vi "DEMO_01_SER-2014.vi"() -> ()   [LabVIEW 2014]
uses:
  <vilib>/Instr/_visa.llb/VISA Configure Serial Port (Instr).vi
panel:
  in  "开闭环":u16(ring) items=["  开环", "  闭环"]
  in  "通道":enum16{"  一路", "  二路", "  三路"}(ring)
  in  "发送数据":dbl
  out "添加的数组":i32[](array[numeric])
  out "抑或后的数据值":u8
  in  "stop":bool
  in  "退出":bool
  in  "发送":bool
  in  "上位机控制":bool
  in  "VISA资源名称":refnum<visa-resource-name>="COM1"
  in  "波特率":u32(ring)=9600 items=["75"=75, "110"=110, "134"=134, "150"=150, "300"=300, "600"=600, "1200"=1200, "1800"=1800, "2400"=2400, "4800"=4800, "7200"=7200, "9600"=9600, "14400"=14400, "19200"=19200, "28800"=28800, "38400"=38400, "56000"=56000, "57600"=57600, "115200"=115200, "128000"=128000, "230400"=230400]
  in  "奇偶":enum16{"None", "Odd", "Even", "Mark", "Space"}(ring) caption="校验"
  # "哈尔滨芯明天科技labview例程发送单点数据"
  # "测试的数组"
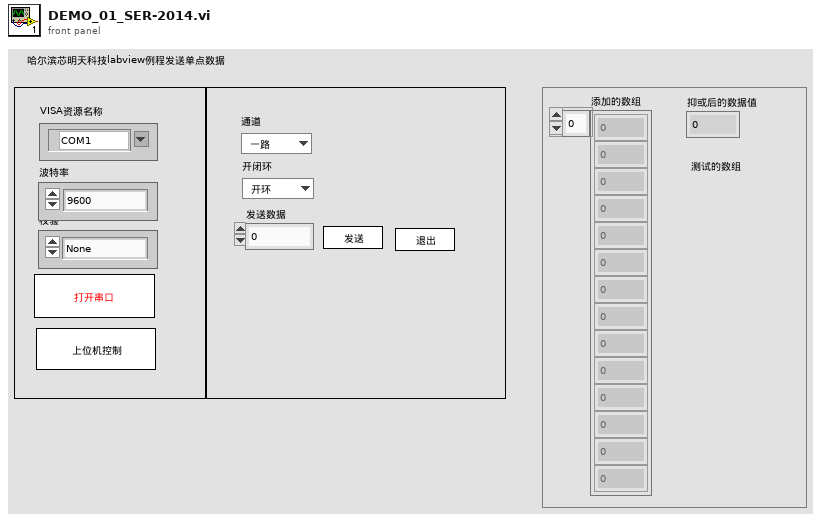
[diagram p1: front panel]
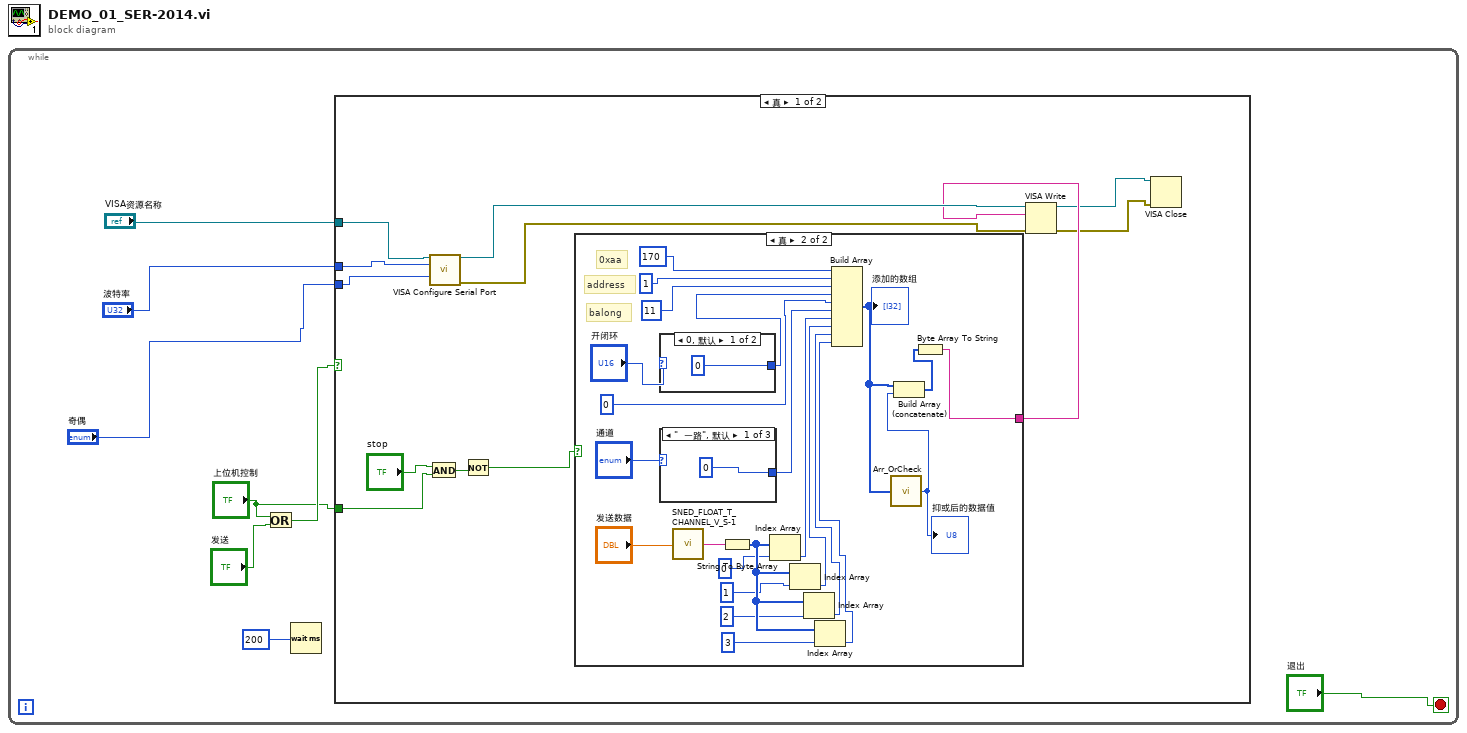
[diagram p0: block diagram]
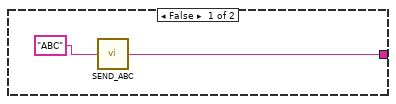
[diagram p2: hidden frame]
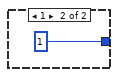
[diagram p3: hidden frame]
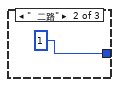
[diagram p4: hidden frame]
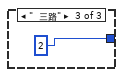
[diagram p5: hidden frame]
diagram:
  n1 = while {
    stop <- "退出" stop-if-true
    n2 = Or(x="上位机控制", y="发送") -> (x .or. y?=w6:bool)
    n3 = Wait (ms)(milliseconds to wait=200) -> ()  [unwired: 1 out]
    n4 = case shown="真" w6 {
      tunnel: "VISA资源名称" -> [w20 _]
      tunnel: "波特率" -> [w19 _]
      tunnel: "奇偶" -> [w18 _]
      tunnel: "上位机控制" -> [w13 _]
      frame True {
        n5 = And(x="stop", y=w13) -> (x .and. y?=w12:bool)
        n6 = call-poly "VISA Configure Serial Port"("VISA resource name"=w20, "baud rate (9600)"=w19, "parity (0:none)"=w18) -> ("VISA resource name out"=w17:refnum<visa-resource-name>, "error out"=w16:errorcluster)  [unwired: 11 in]
        n7 = Not(x=w12) -> (.not. x?=w11:bool)
        n8 = case shown="真" w11 {
          tunnel: [w21 w25] -> w15
          frame False {
            n9 = call "SEND_ABC.vi"("SEND_ARR"="ABC") -> ("SEND_CHR"=w21:string)
          }
          frame True {
            # "balong"
            # "address"
            # "0xaa"
            n10 = case shown="0, 默认" "开闭环" {
              tunnel: [0 1] -> w33
              frame 0, Default {
              }
              frame 1 {
              }
            }
            n11 = case shown="\"  一路\", 默认" "通道" {
              tunnel: [0 1 2] -> w31
              frame "  一路", Default {
              }
              frame "  二路" {
              }
              frame "  三路" {
              }
            }
            n12 = call "SNED_FLOAT_T_CHANNEL_V_S-1.vi"("数据"="发送数据") -> ("字符串"=w42:string)
            n13 = String To Byte Array(string=w42) -> (unsigned byte array=w41:u8[])
            n14 = Index Array(array=w41, index=0) -> (element=w30:u8)
            n15 = Index Array(array=w41, index=1) -> (element=w29:u8)
            n16 = Index Array(array=w41, index=2) -> (element=w28:u8)
            n17 = Index Array(array=w41, index=3) -> (element=w27:u8)
            n18 = Build Array(170, 1, 11, w33, 0, w31, w30, w29, w28, w27) -> (w23:i32[])
            "添加的数组" <- w23
            n19 = call "Arr_OrCheck.vi"("数组"=w23) -> ("抑或的数据值"=w24:u8)
            "抑或后的数据值" <- w24
            n20 = Build Array (concatenate)(w23, w24) -> (w26:i32[])
            n21 = Byte Array To String(unsigned byte array=w26) -> (string=w25:string)
          }
        }
        n22 = VISA Write(VISA resource name=w17, write buffer=w15, error in (no error)=w16) -> (VISA resource name out=w10:refnum<visa-resource-name>, error out=w9:errorcluster)  [unwired: 1 out]
        n23 = VISA Close(VISA resource name=w10, error in (no error)=w9) -> ()  [unwired: 1 out]
      }
      frame False {
      }
    }
  }
